vi "Init.vi"(8 "error in (no error)":errorcluster, 10 "Msg Handlers":refnum<queue>, 11 "Send Queue":refnum<queue>) -> (0 "error out":errorcluster, 3 "TCPMessageService out":refnum<class "TCPMessageAPI.lvclass">)   [LabVIEW 2020, in "Vecto.lvlib" / "TCPMessageAPI.lvclass"]
uses:
  TCPMessageAPI.lvclass
  proto/TcpPayload/Data.ctl
  TCPMessageHandler/TCPMessageHandler.lvclass
  TCPMessageAPI.lvclass/TCPMessageAPI.ctl
  proto/TcpPayload/TcpPayload.lvlib
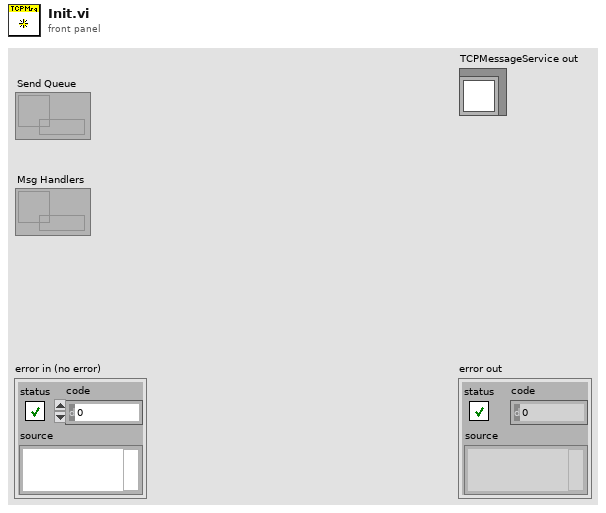
[diagram p1: front panel]
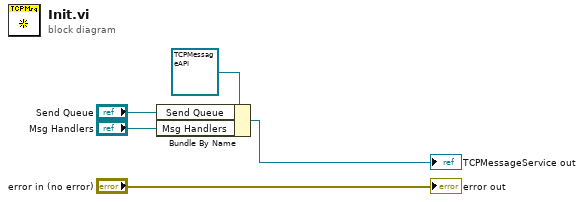
[diagram p0: block diagram]
diagram:
  n1 = Bundle By Name(cluster=refnum<class "TCPMessageAPI.lvclass"> refnum ("TCPMessageService in"), "Send Queue"="Send Queue", "Msg Handlers"="Msg Handlers") -> (→"TCPMessageService out":refnum<class "TCPMessageAPI.lvclass">)
  "error out" <- "error in (no error)"
